vi "FindFirstLetter.vi"(10 "String Array":string[](array[string])) -> (1 "Found?":bool, 2 "Index":i32, 3 "Character":string)   [LabVIEW 2020, in "Parse.Paths.lvclass"]
uses:
  Parse.Paths.lvclass
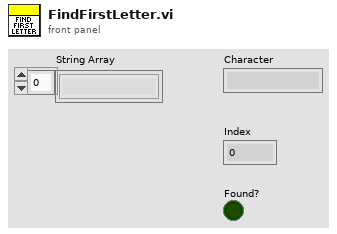
[diagram p1: front panel]
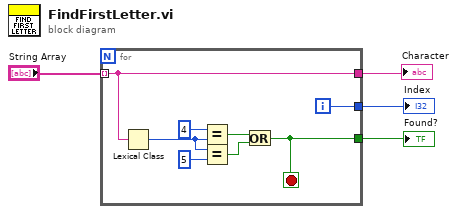
[diagram p0: block diagram]
diagram:
  n1 = for {
    tunnel: "String Array" -> [w6] mode=indexing
    tunnel: [w7] -> w3
    tunnel: [w6] -> w2
    tunnel: [w5] -> w1
    i -> [w7]
    stop <- w5 stop-if-true
    n2 = Lexical Class(1:w6) -> (0:w11:i16)
    n3 = Equal?(x=i16 4, y=w11) -> (x = y?=w9:bool)
    n4 = Equal?(x=w11, y=i16 5) -> (x = y?=w8:bool)
    n5 = Or(x=w9, y=w8) -> (x .or. y?=w5:bool)
  }
  "Index" <- w3
  "Character" <- w2
  "Found?" <- w1
